vi "Memory.Pointer.Copy.Unsafe.vi"(8 "error in (no error)":errorcluster, 9 "bytes to copy":u64 format="%08x bytes", 10 "dst pointer in":refnum<class "Memory.Pointer.lvclass">, 11 "src pointer in":refnum<class "Memory.Pointer.lvclass">) -> (0 "error out":errorcluster, 1 "bytes to copy":u64 format="%08x bytes", 2 "dst pointer out":refnum<class "Memory.Pointer.lvclass">, 3 "src pointer out":refnum<class "Memory.Pointer.lvclass">)   [LabVIEW 2016, in "Memory Manager.lvlib" / "Memory.Pointer.lvclass"]
uses:
  Memory.Pointer.lvclass
  Memory.Pointer.lvclass/Memory.Pointer.ctl
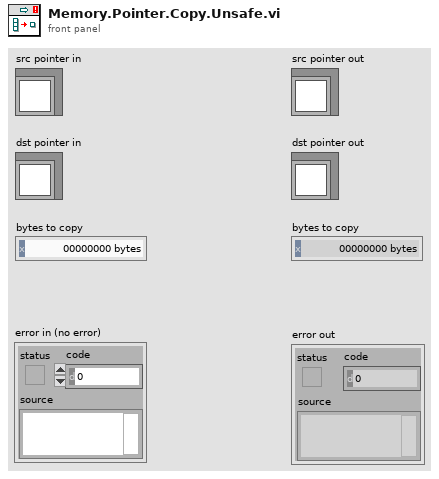
[diagram p1: front panel]
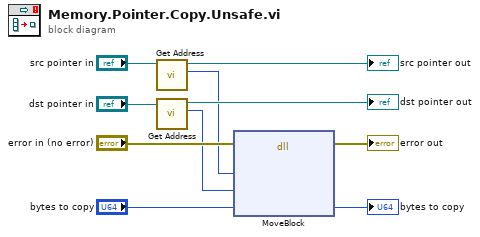
[diagram p0: block diagram]
diagram:
  n1 = call "Get Address.vi"("Pointer in"="src pointer in") -> ("address"=w3:u64, "Pointer out"=→"src pointer out":refnum<class "Memory.Pointer.lvclass">)  [unwired: 8 in, 1 out]
  n2 = call "Get Address.vi"("Pointer in"="dst pointer in") -> ("address"=w4:u64, "Pointer out"=→"dst pointer out":refnum<class "Memory.Pointer.lvclass">)  [unwired: 8 in, 1 out]
  n3 = dll-call lib="LabVIEW" fn="MoveBlock"(error in="error in (no error)", "src"=w3, "dst"=w4, "size"="bytes to copy") -> (error out=→"error out":errorcluster, "size"=→"bytes to copy":u64)  [unwired: 5 in, 1 out]
